vi "fpga_96ch-Super_mux.vi"(1 "12 8Ch-timestamp groups":T2) -> (0 "All Ch Timestamps":T1)   [LabVIEW 2011]
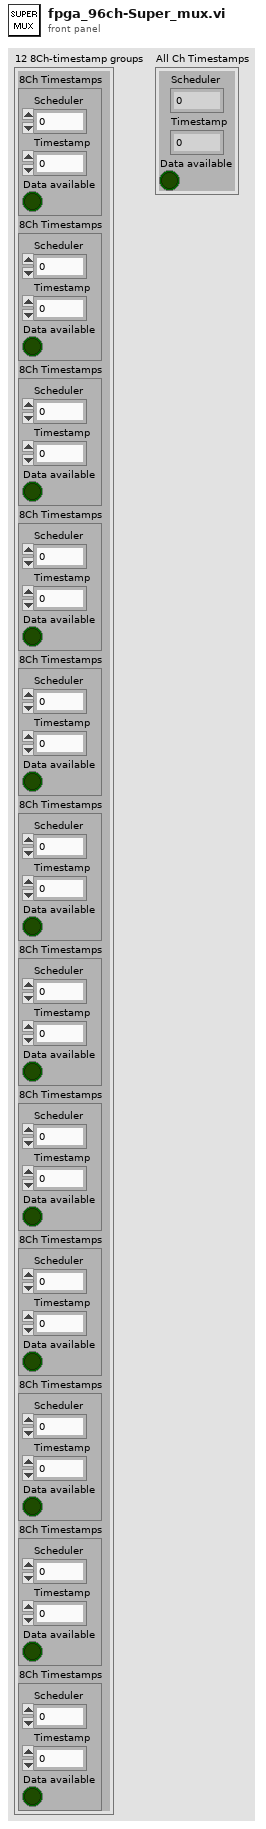
[diagram p1: front panel]
types:
  T1 = cluster{"Scheduler":u8, "Timestamp":u32, "Data available":bool}
  T2 = cluster{"8Ch Timestamps":cluster{"Scheduler":u8, "Timestamp":u32, "Data available":bool}, "8Ch Timestamps":cluster{"Scheduler":u8, "Timestamp":u32, "Data available":bool}, "8Ch Timestamps":cluster{"Scheduler":u8, "Timestamp":u32, "Data available":bool}, "8Ch Timestamps":cluster{"Scheduler":u8, "Timestamp":u32, "Data available":bool}, "8Ch Timestamps":cluster{"Scheduler":u8, "Timestamp":u32, "Data available":bool}, "8Ch Timestamps":cluster{"Scheduler":u8, "Timestamp":u32, "Data available":bool}, "8Ch Timestamps":cluster{"Scheduler":u8, "Timestamp":u32, "Data available":bool}, "8Ch Timestamps":cluster{"Scheduler":u8, "Timestamp":u32, "Data available":bool}, "8Ch Timestamps":cluster{"Scheduler":u8, "Timestamp":u32, "Data available":bool}, "8Ch Timestamps":cluster{"Scheduler":u8, "Timestamp":u32, "Data available":bool}, "8Ch Timestamps":cluster{"Scheduler":u8, "Timestamp":u32, "Data available":bool}, "8Ch Timestamps":cluster{"Scheduler":u8, "Timestamp":u32, "Data available":bool}}
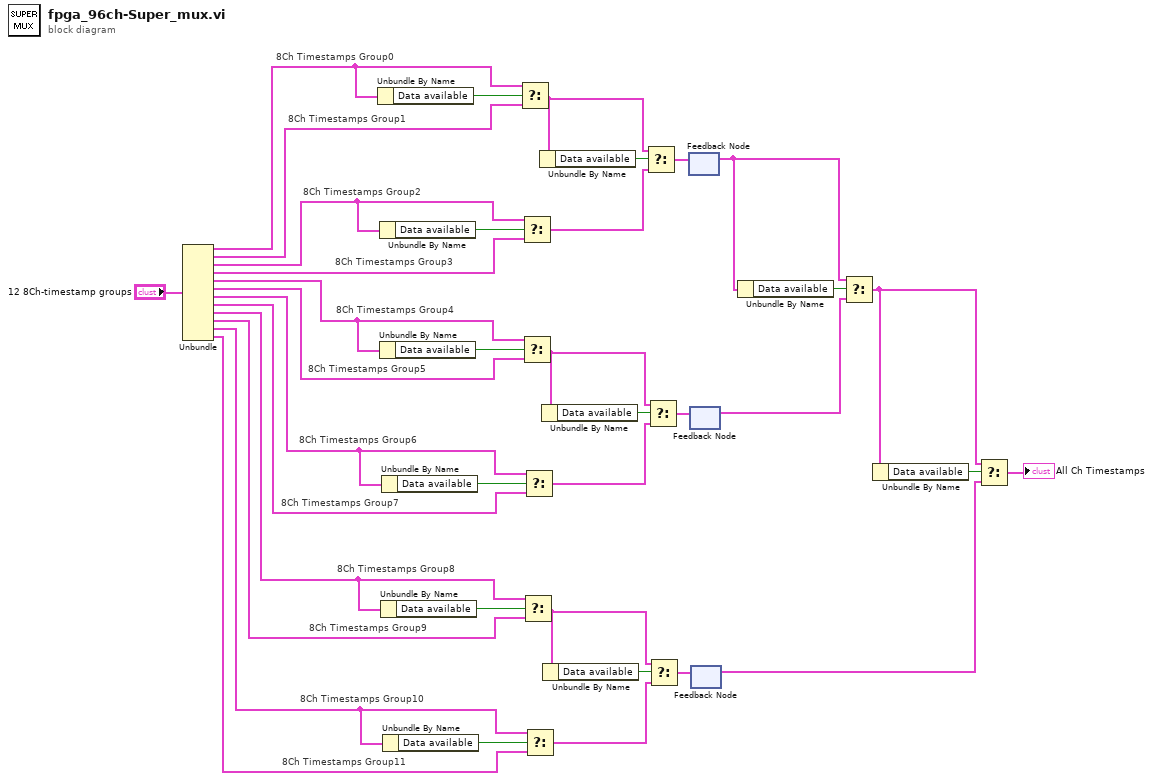
[diagram p0: block diagram]
diagram:
  # "8Ch Timestamps Group11"
  # "8Ch Timestamps Group10"
  # "8Ch Timestamps Group9"
  # "8Ch Timestamps Group8"
  # "8Ch Timestamps Group7"
  # "8Ch Timestamps Group6"
  # "8Ch Timestamps Group5"
  # "8Ch Timestamps Group4"
  # "8Ch Timestamps Group3"
  # "8Ch Timestamps Group2"
  # "8Ch Timestamps Group1"
  # "8Ch Timestamps Group0"
  n1 = Unbundle("12 8Ch-timestamp groups") -> ("8Ch Timestamps"=w25:T1, "8Ch Timestamps"=w24:T1, "8Ch Timestamps"=w23:T1, "8Ch Timestamps"=w22:T1, "8Ch Timestamps"=w21:T1, "8Ch Timestamps"=w20:T1, "8Ch Timestamps"=w19:T1, "8Ch Timestamps"=w18:T1, "8Ch Timestamps"=w8:T1, "8Ch Timestamps"=w7:T1, "8Ch Timestamps"=w6:T1, "8Ch Timestamps"=w5:T1)
  n2 = Unbundle By Name(w25) -> ("Data available"=w38:bool)
  n3 = Unbundle By Name(w23) -> ("Data available"=w37:bool)
  n4 = Unbundle By Name(w21) -> ("Data available"=w33:bool)
  n5 = Unbundle By Name(w8) -> ("Data available"=w14:bool)
  n6 = Unbundle By Name(w19) -> ("Data available"=w32:bool)
  n7 = Unbundle By Name(w6) -> ("Data available"=w13:bool)
  n8 = Select(t=w25, s=w38, f=w24) -> (s? t:f=w36:T1)
  n9 = Select(t=w23, s=w37, f=w22) -> (s? t:f=w35:T1)
  n10 = Select(t=w21, s=w33, f=w20) -> (s? t:f=w31:T1)
  n11 = Select(t=w8, s=w14, f=w7) -> (s? t:f=w12:T1)
  n12 = Select(t=w19, s=w32, f=w18) -> (s? t:f=w30:T1)
  n13 = Select(t=w6, s=w13, f=w5) -> (s? t:f=w11:T1)
  n14 = Unbundle By Name(w36) -> ("Data available"=w34:bool)
  n15 = Unbundle By Name(w31) -> ("Data available"=w29:bool)
  n16 = Unbundle By Name(w12) -> ("Data available"=w10:bool)
  n17 = Select(t=w36, s=w34, f=w35) -> (s? t:f=w27:T1)
  n18 = Select(t=w31, s=w29, f=w30) -> (s? t:f=w28:T1)
  n19 = Select(t=w12, s=w10, f=w11) -> (s? t:f=w9:T1)
  n20 = feedback-in #1(w27) -> ()
  n21 = feedback #1() -> (w17:T1)  [unwired: 1 in]
  n22 = feedback-in #2(w28) -> ()
  n23 = feedback #2() -> (w16:T1)  [unwired: 1 in]
  n24 = feedback #3() -> (w3:T1)  [unwired: 1 in]
  n25 = feedback-in #3(w9) -> ()
  n26 = Unbundle By Name(w17) -> ("Data available"=w26:bool)
  n27 = Select(t=w17, s=w26, f=w16) -> (s? t:f=w4:T1)
  n28 = Unbundle By Name(w4) -> ("Data available"=w2:bool)
  n29 = Select(t=w4, s=w2, f=w3) -> (s? t:f=→"All Ch Timestamps":T1)
